vi "Write Repo_Name.vi"(8 "error in (no error)":errorcluster, 10 "Repo_Name":string, 11 "VIP Publish in":refnum<class "VIP Publish.lvclass">) -> (0 "error out":errorcluster, 3 "VIP Publish out":refnum<class "VIP Publish.lvclass">)   [LabVIEW 2014, in "VIP Publish.lvclass"]
uses:
  VIP Publish.lvclass
  VIP Publish.lvclass/VIP Publish.ctl
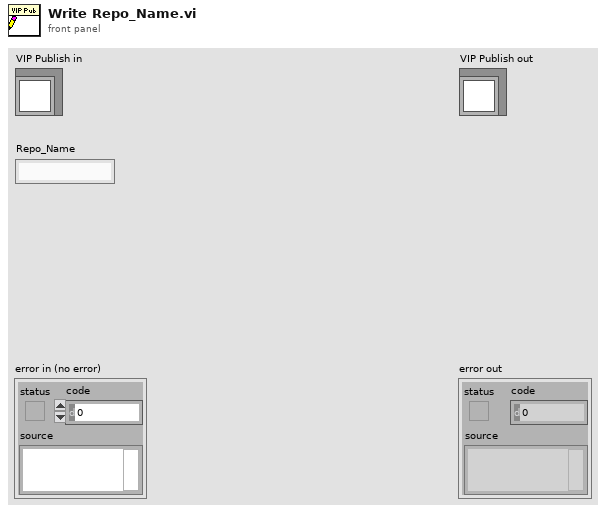
[diagram p1: front panel]
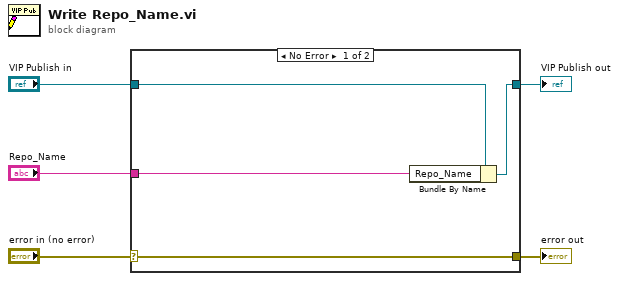
[diagram p0: block diagram]
diagram:
  n1 = case shown="No Error" "error in (no error)" {
    selector: "error in (no error)" -> [w9 w10]
    tunnel: [w9 w10] -> w4
    tunnel: [w7 w11] -> w2
    tunnel: "VIP Publish in" -> [w8 w11]
    tunnel: "Repo_Name" -> [w6 _]
    frame No Error {
      n2 = Bundle By Name(cluster=w8, "Repo_Name"=w6) -> (w7:refnum<class "VIP Publish.lvclass">)
    }
    frame Error {
    }
  }
  "error out" <- w4
  "VIP Publish out" <- w2
